vi "file ps.vi"(11 "field":T1) -> (3 "field out":T1)   [LabVIEW 2012, in "LightPipes.lvlib"]
doc: "__declspec(dllexport) void file_ps (FIELD* field );"
uses:
  LightPipes.lvlib
  Lightpipes.dll
panel:
  out "error out":errorcluster
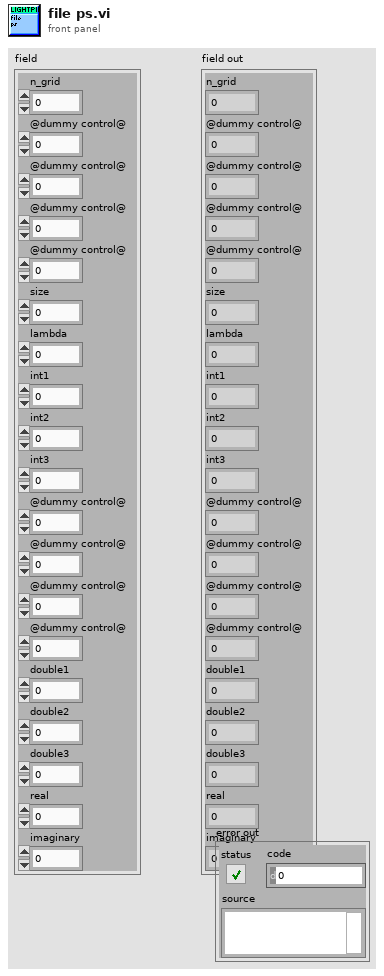
[diagram p1: front panel]
types:
  T1 = cluster{"n_grid":i32, "@dummy control@":i8, "@dummy control@":i8, "@dummy control@":i8, "@dummy control@":i8, "size":dbl, "lambda":dbl, "int1":i32, "int2":i32, "int3":i32, "@dummy control@":i8, "@dummy control@":i8, "@dummy control@":i8, "@dummy control@":i8, "double1":dbl, "double2":dbl, "double3":dbl, "real":u32, "imaginary":u32}
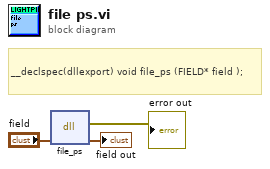
[diagram p0: block diagram]
diagram:
  # "__declspec(dllexport) void file_ps (FIELD* field );"
  n1 = dll-call lib="C:/Users/Tri/Documents/Gerchberg/LightPipes.*" fn="file_ps"("field"="field") -> (error out=→"error out":errorcluster, "field"=→"field out":T1)  [unwired: 4 in, 1 out]
